vi "OpenConnection.vi"(8 "error in (no error)":errorcluster, 11 "Modbus In":refnum<class "Modbus.lvclass">) -> (0 "error out":errorcluster, 3 "Modbus Out":refnum<class "Modbus.lvclass">)   [LabVIEW 2019, in "Modbus.lvclass"]
uses:
  Modbus.lvclass
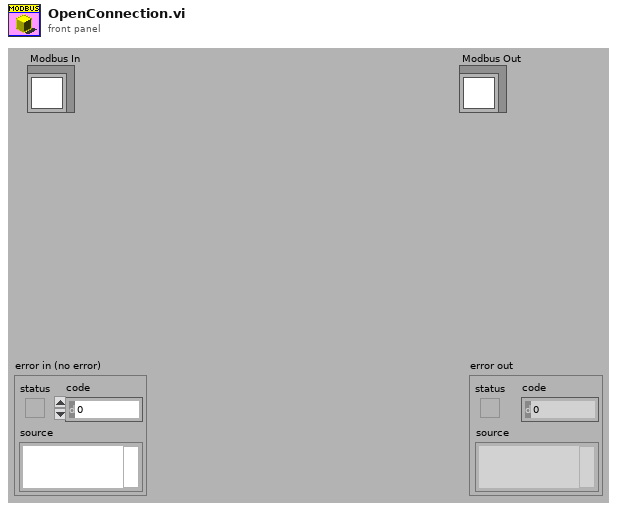
[diagram p1: front panel]
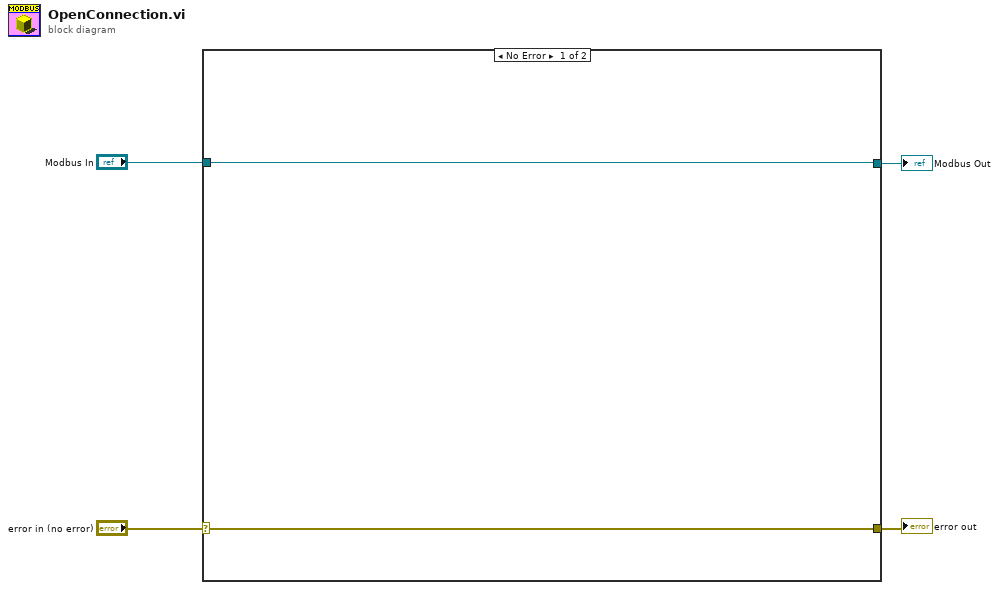
[diagram p0: block diagram]
diagram:
  n1 = case shown="No Error" "error in (no error)" {
    selector: "error in (no error)" -> [w6 w8]
    tunnel: [w6 w8] -> w3
    tunnel: [w5 w7] -> w1
    tunnel: "Modbus In" -> [w5 w7]
    frame No Error {
    }
    frame Error {
    }
  }
  "error out" <- w3
  "Modbus Out" <- w1
